vi "Set ByRef (Unnamed SEQ).vi"(8 "error in (no error)":errorcluster, 10 "Int":i32, 11 "Numeric in":refnum<class "Numeric Test Object.lvclass">) -> (0 "error out":errorcluster, 3 "Numeric out":refnum<class "Numeric Test Object.lvclass">)   [LabVIEW 2009, in "Numeric Test Object.lvclass"]
doc: "Sets the by-ref data held by the unnamed single element queue."
uses:
  Numeric Test Object.lvclass
  Numeric Test Object.lvclass/Numeric Test Object.ctl
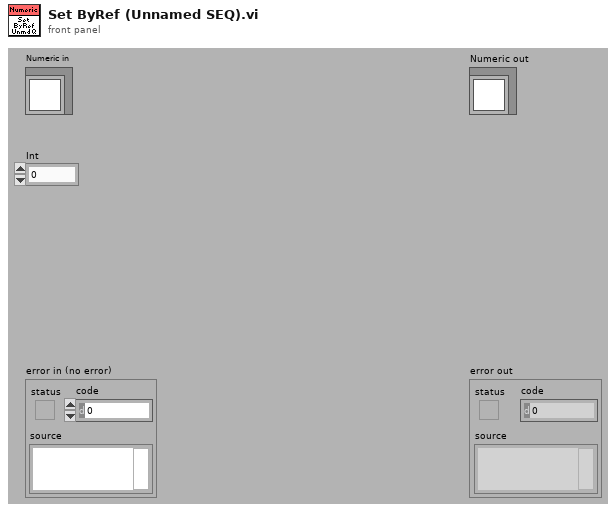
[diagram p1: front panel]
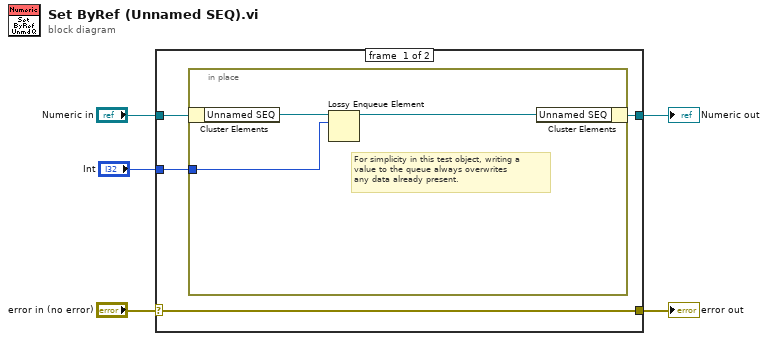
[diagram p0: block diagram]
diagram:
  n1 = case shown="No Error" "error in (no error)" {
    selector: "error in (no error)" -> [w9 w13]
    tunnel: [w9 w13] -> w4
    tunnel: [w7 w14] -> w2
    tunnel: "Numeric in" -> [w8 w14]
    tunnel: "Int" -> [w6 _]
    frame #0 {
      n2 = in-place {
        in-place-border: w6 -> [w10]
        # "For simplicity in this test object, writing a\nvalue to the queue always overwrites\nany data already present."
        n3 = in-place-cluster #1(w8) -> ("Unnamed SEQ"=w12:refnum<queue>)
        n4 = Lossy Enqueue Element(queue=w12, element=w10) -> (queue out=w11:refnum<queue>)  [unwired: 1 in, 3 out]
        n5 = in-place-cluster #1("Unnamed SEQ"=w11) -> (w7:refnum<class "Numeric Test Object.lvclass">)
      }
    }
    frame #1 {
    }
  }
  "error out" <- w4
  "Numeric out" <- w2
